vi "Read Write_RIO to Dashboard controls.vi"(10 "Read(F) Write(T)":bool, 11 "Data In":T1) -> (3 "Data Out":T1)   [LabVIEW 2017]
uses:
  TypeDefs/Cluster_RIO to DashBoard Controls.ctl
  <vilib>/Rock Robotics/Network Tables/NT Read Numeric Array.vi
  <vilib>/Rock Robotics/Network Tables/NT Write Numeric Array.vi
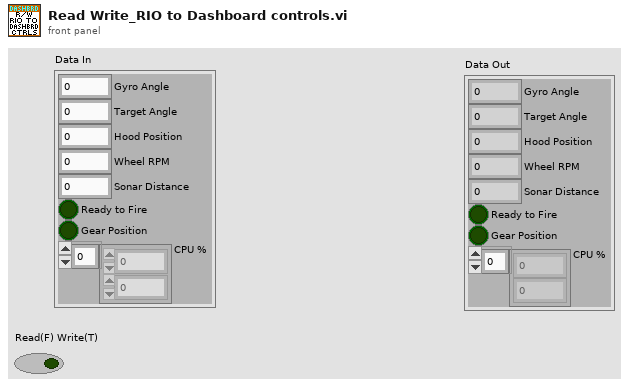
[diagram p1: front panel]
types:
  T1 = typedef "Cluster_RIO to DashBoard Controls.ctl" = cluster{"Gyro Angle":dbl, "Target Angle":dbl, "Hood Position":dbl, "Wheel RPM":dbl, "Sonar Distance":dbl, "Ready to Fire":bool, "Gear Position":bool, "CPU %":dbl[]}
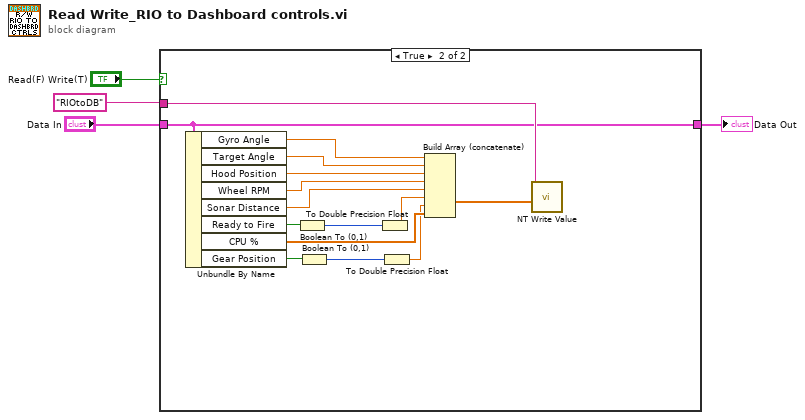
[diagram p0: block diagram]
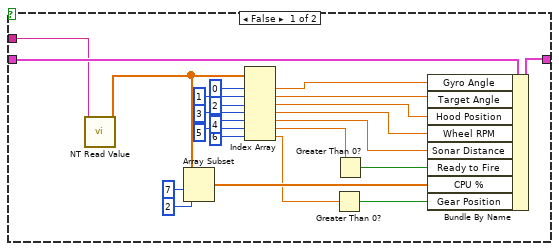
[diagram p2: hidden frame]
diagram:
  n1 = case shown="True" "Read(F) Write(T)" {
    tunnel: [w26 w41] -> w3
    tunnel: "Data In" -> [w27 w41]
    tunnel: "RIOtoDB" ("string") -> [w25 w42]
    frame False {
      n2 = call-poly <vilib>:"NT Read Value.vi"("Name"=w25) -> ("Numeric Array"=w11:dbl[])  [unwired: 9 in, 1 out]
      n3 = Array Subset(array=w11, index=7, length=2) -> (w10:dbl[])
      n4 = Index Array(array=w11, index #1=0 ("index"), index #2=1 ("index"), index #3=2 ("index"), index #4=3 ("index"), index #5=4 ("index"), index #6=5 ("index"), index #7=6 ("index")) -> (element #1=w24:dbl, element #2=w23:dbl, element #3=w22:dbl, element #4=w21:dbl, element #5=w20:dbl, element #6=w19:dbl, element #7=w6:dbl)
      n5 = Greater Than 0?(x=w6) -> (x > 0?=w5:bool)
      n6 = Greater Than 0?(x=w19) -> (x > 0?=w18:bool)
      n7 = Bundle By Name(cluster=w27, "Gyro Angle"=w24, "Target Angle"=w23, "Hood Position"=w22, "Wheel RPM"=w21, "Sonar Distance"=w20, "Ready to Fire"=w18, "CPU %"=w10, "Gear Position"=w5) -> (w26:T1)
    }
    frame True {
      n8 = Unbundle By Name(w41) -> ("Gyro Angle"=w40:dbl, "Target Angle"=w39:dbl, "Hood Position"=w38:dbl, "Wheel RPM"=w37:dbl, "Sonar Distance"=w36:dbl, "Ready to Fire"=w35:bool, "CPU %"=w29:dbl[], "Gear Position"=w30:bool)
      n9 = Boolean To (0,1)(Boolean=w35) -> (0, 1=w34:i16)
      n10 = Boolean To (0,1)(Boolean=w30) -> (0, 1=w31:i16)
      n11 = To Double Precision Float(number=w34) -> (double precision float=w33:dbl)
      n12 = To Double Precision Float(number=w31) -> (double precision float=w28:dbl)
      n13 = Build Array (concatenate)(w40, w39, w38, w37, w36, w33, w28, w29) -> (w32:dbl[])
      n14 = call-poly <vilib>:"NT Write Value.vi"("Numeric Array"=w32, "Name"=w42) -> ()  [unwired: 9 in, 1 out]
    }
  }
  "Data Out" <- w3
